vi "Real FFT(half complex).vi"(0 "X":dbl[](array[numeric]) format="%0.2f") -> (1 "FFT {X}":dbl[](array[numeric]) format="%0.2f", 2 "error":i32)   [LabVIEW 2024, in "NI_AALPro.lvlib"]
doc: "Computes the Real Fast Fourier Transform (FFT) or the Real Discrete Fourier Transform (DFT) of the input sequence <B>X</B>."
uses:
  NI_AALPro.lvlib
  <resource>/lvanlys.dll
panel:
  # "Real (half complex) FFT"
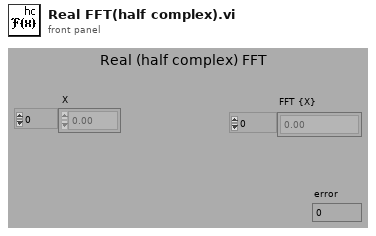
[diagram p1: front panel]
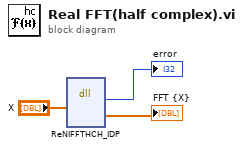
[diagram p0: block diagram]
diagram:
  n1 = dll-call lib="C:/Program Files (x86)/National Instruments/LabVIEW 2024/resource/lvanlys.*" fn="ReNIFFTHCH_IDP"("xH"="X") -> ("return type"=→"error":i32, "yH"=→"FFT {X}":dbl[])  [unwired: 7 in, 2 out]
